vi "PAN_BuildSlowCmdID.vi"(8 "error in (no error)":errorcluster, 9 "Command":string, 10 "caller":string) -> (0 "error out":errorcluster, 2 "cmdID":string)   [LabVIEW 2016]
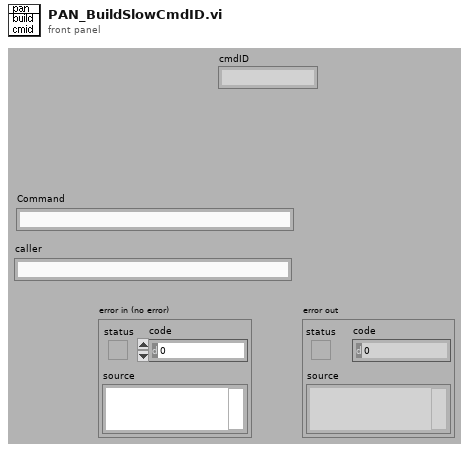
[diagram p1: front panel]
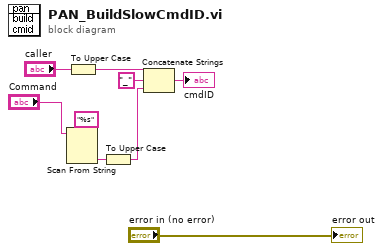
[diagram p0: block diagram]
diagram:
  n1 = Scan From String(format string="%s", input string="Command") -> (output 1=w3:string)  [unwired: 2 in, 4 out]
  n2 = To Upper Case(1:"caller") -> (0:w1:string)
  n3 = To Upper Case(1:w3) -> (0:w2:string)
  n4 = Concatenate Strings(w1, "_" ("string"), w2) -> (→"cmdID":string)
  "error out" <- "error in (no error)"
